vi "Vaciado de Tanques.vi"() -> ()   [LabVIEW 2019]
panel:
  out "Tank":dbl(slide) scale=0.0..10.0
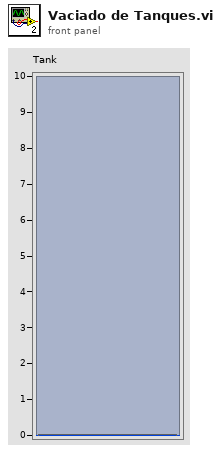
[diagram p1: front panel]
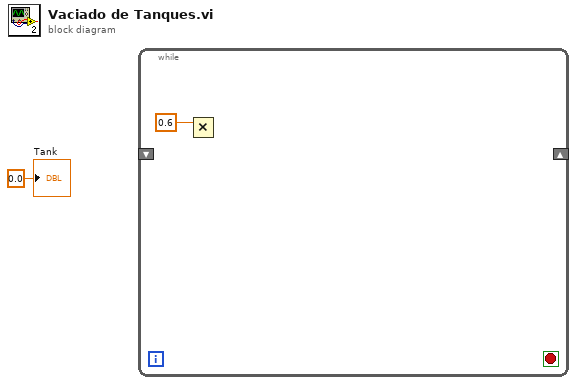
[diagram p0: block diagram]
diagram:
  n1 = while {
    shift-right: _ -> [_]
    shift-left: _ -> [_]
    stop <- _ stop-if-true
    n2 = Multiply(x=0.6) -> ()  [unwired: 1 in, 1 out]
  }
  "Tank" <- 0.0 ("Tank")
